vi "create ws.vi"() -> ()   [LabVIEW 2020]
uses:
  <resource>/Framework/Providers/ws_project_provider/common/Web Service VI.ctl
  <resource>/Framework/Providers/ws_project_provider/common/Web Service VI Type.ctl
  <resource>/Framework/Providers/ws_project_provider/common/Web Service VI Method.ctl
  <resource>/Framework/Providers/ws_project_provider/common/Web Service VI Output Type.ctl
  <resource>/Framework/Providers/ws_project_provider/common/Web Service VI Output Format.ctl
  <resource>/Framework/Providers/ws_project_provider/common/NI Web Service Provider.lvlib
panel:
  out "Error Out 3":errorcluster
  out "Web service VI":T1={"item"=0, "item ID"="", "Web Service VI Type"=enum."<DUMMY>", "Method"=enum."<DUMMY>", "Load at startup"=FALSE, "Keep in memory"=FALSE, "Output type"=enum."Terminal", "Output format"=enum."XML", "Use headers"=FALSE, "Buffered"=FALSE, "Require API key"=FALSE, "Permissions"="", "Standard URL"=FALSE, "Include VI name in URL"=FALSE, "Custom URL"="", "Required Privilege"=""}
  out "output cluster":T1={"item"=0, "item ID"="", "Web Service VI Type"=enum."<DUMMY>", "Method"=enum."<DUMMY>", "Load at startup"=FALSE, "Keep in memory"=FALSE, "Output type"=enum."Terminal", "Output format"=enum."XML", "Use headers"=FALSE, "Buffered"=FALSE, "Require API key"=FALSE, "Permissions"="", "Standard URL"=FALSE, "Include VI name in URL"=FALSE, "Custom URL"="", "Required Privilege"=""}
  out "Error Out":errorcluster
  out "NIIM":T6
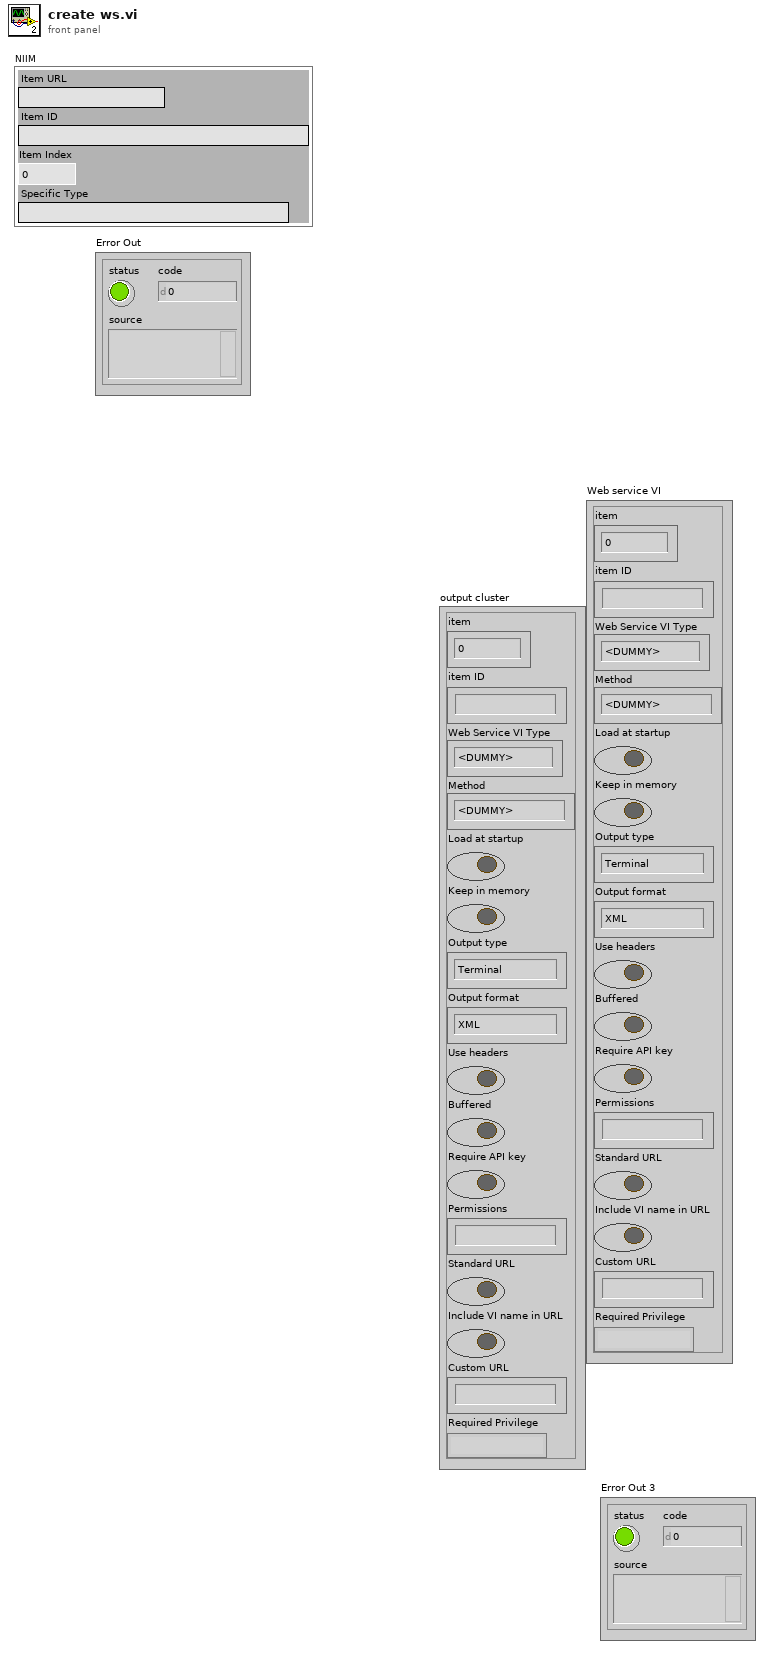
[diagram p1: front panel]
types:
  T1 = typedef "NI Web Service Provider.lvlib/Web Service VI.ctl" = cluster{"item":u64, "item ID":string, "Web Service VI Type":T2, "Method":T3, "Load at startup":bool, "Keep in memory":bool, "Output type":T4, "Output format":T5, "Use headers":bool, "Buffered":bool, "Require API key":bool, "Permissions":string, "Standard URL":bool, "Include VI name in URL":bool, "Custom URL":string, "Required Privilege":string}
  T2 = typedef "NI Web Service Provider.lvlib/Web Service VI Type.ctl" = enum16{"<DUMMY>", "Web Method", "Auxiliary", "Internal", "Content"}
  T3 = typedef "NI Web Service Provider.lvlib/Web Service VI Method.ctl" = enum16{"<DUMMY>", "GET", "PUT", "POST", "DELETE", "OPTIONS", "HEAD", "TRACE"}
  T4 = typedef "NI Web Service Provider.lvlib/Web Service VI Output Type.ctl" = enum16{"Terminal", "Stream"}
  T5 = typedef "NI Web Service Provider.lvlib/Web Service VI Output Format.ctl" = enum16{"<DUMMY>", "Text", "XML", "HTML", "JSON"}
  T6 = cluster{"Item URL":string, "Item ID":string, "Item Index":i32, "Specific Type":string}
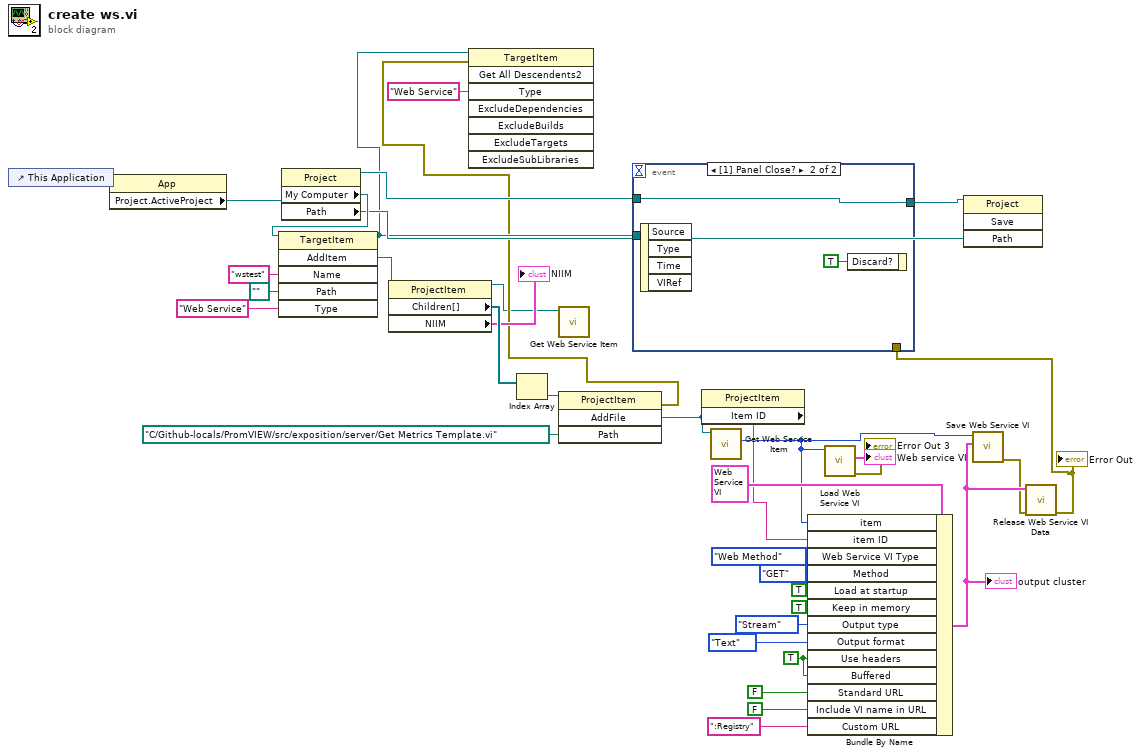
[diagram p0: block diagram]
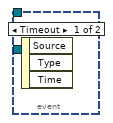
[diagram p2: hidden frame]
diagram:
  w17 = TRUE ("Use headers")
  n1 = control-ref of="This Application"() -> (w36:refnum<vi>)
  n2 = property class="App"(reference=w36) -> ("Project.ActiveProject"=w35:refnum<vi>)  [unwired: 1 in, 2 out]
  n3 = property class="Project"(reference=w35) -> (reference out=w30:refnum<vi>, "My Computer"=w34:refnum<vi>, "Path"=w32:path)  [unwired: 1 in, 1 out]
  n4 = invoke class="TargetItem" method="AddItem"(reference=w34, "Name"="wstest", "Path"=path "", "Type"="Web Service") -> (reference out=w13:refnum<vi>, "AddItem"=w29:refnum<vi>)  [unwired: 2 in, 4 out]
  n5 = property class="ProjectItem"(reference=w29) -> (reference out=w10:refnum<vi>, "Children[]"=w28:refnum<vi>[], "NIIM"=→"NIIM":T6)  [unwired: 1 in, 1 out]
  n6 = Index Array(array=w28) -> (element=w27:refnum<vi>)  [unwired: 1 in]
  n7 = call <resource>:"Get Web Service Item.vi"("Web service project item"=w10) -> ()  [unwired: 8 in, 3 out]
  n8 = invoke class="ProjectItem" method="AddFile"(reference=w27, "Path"=path "C:/Github-locals/PromVIEW/src/exposition/server/Get Metrics Template.vi") -> (error out=w11:errorcluster, "AddFile"=w9:refnum<vi>)  [unwired: 2 in, 2 out]
  n9 = invoke class="TargetItem" method="Get All Descendents2"(reference=w13, error in=w11, "Type"="Web Service") -> ()  [unwired: 5 in, 8 out]
  n10 = property class="ProjectItem"(reference=w9) -> ("Item ID"=w8:string)  [unwired: 1 in, 2 out]
  n11 = call <resource>:"Get Web Service Item.vi"("Web service project item"=w9) -> ("Web service item"=w5:u64)  [unwired: 8 in, 2 out]
  n12 = Bundle By Name(cluster=T1 {"item"=0, "item ID"="", "Web Service VI Type"=enum."<DUMMY>", "Method"=enum."<DUMMY>", "Load at startup"=FALSE, "Keep in memory"=FALSE, "Output type"=enum."Terminal", "Output format"=enum."XML", "Use headers"=FALSE, "Buffered"=FALSE, "Require API key"=FALSE, "Permissions"="", "Standard URL"=FALSE, "Include VI name in URL"=FALSE, "Custom URL"="", "Required Privilege"=""} ("Web service VI"), "item"=w5, "item ID"=w8, "Web Service VI Type"=Web_Service_VI_Type."Web Method", "Method"=Web_Service_VI_Method."GET", "Load at startup"=TRUE, "Keep in memory"=TRUE, "Output type"=Web_Service_VI_Output_Type."Stream", "Output format"=Web_Service_VI_Output_Format."Text", "Use headers"=w17, "Buffered"=w17, "Standard URL"=FALSE, "Include VI name in URL"=FALSE, "Custom URL"=":Registry" ("string")) -> (w4:T1)
  "output cluster" <- w4
  n13 = call <resource>:"Load Web Service VI.vi"("Web service item"=w5) -> ("Error Out"=→"Error Out 3":errorcluster, "Web service VI"=→"Web service VI":T1)  [unwired: 8 in, 1 out]
  n14 = call <resource>:"Save Web Service VI.vi"("Web service VI"=w4, "Web service item"=w5) -> ("Error Out"=w3:errorcluster)  [unwired: 7 in, 2 out]
  n15 = call <resource>:"Release Web Service VI Data.vi"("Error In"=w3, "Web service VI"=w4) -> ("Error Out"=w2:errorcluster)  [unwired: 9 in]
  "Error Out" <- w2
  n16 = event shown="[1] Panel Close?" {
    selector: _ -> [_ _]
    dyn-events: _ -> [_ _]
    timeout: _ -> [_ _]
    tunnel: w13 -> [_ _]
    tunnel: [_ w38] -> w31
    tunnel: w30 -> [_ w38]
    tunnel: w2 -> [_ _]
    event Timeout {
      n17 = event-data() -> ()  [unwired: 1 in, 3 out]
    }
    event Panel Close? {
      n18 = event-data() -> ()  [unwired: 1 in, 4 out]
      n19 = event-data("Discard?"=TRUE) -> ()  [unwired: 1 in, 1 out]
    }
  }
  n20 = invoke class="Project" method="Save"(reference=w31, "Path"=w32) -> ()  [unwired: 2 in, 4 out]
